vi "Test Sequence.vi"(0 "FeedBack Channel":string[](array[string])=["fgdgfvcbc", "vnfhgjkn", "21354682"], 1 "Test Name":string, 2 "Steps":T1(array[cluster])) -> (6 "Emergency":bool, 7 "Out":i32, 8 "Condition":bool)   [LabVIEW 2015]
uses:
  <vilib>/Utility/error.llb/whitespace.ctl
  Galobal variable_TI.vi
  Project Setup/Globle Variable/GR_Servo.vi
  <vilib>/Instr/_visa.llb/VISA Configure Serial Port (Instr).vi
panel:
  out "error out 2":errorcluster
  in  "value":bool
  out "read buffer":string
  out "error out":errorcluster
  out "Wait/Poll (ms)":u32
  out "Channels (Out)":i32[](array[numeric])
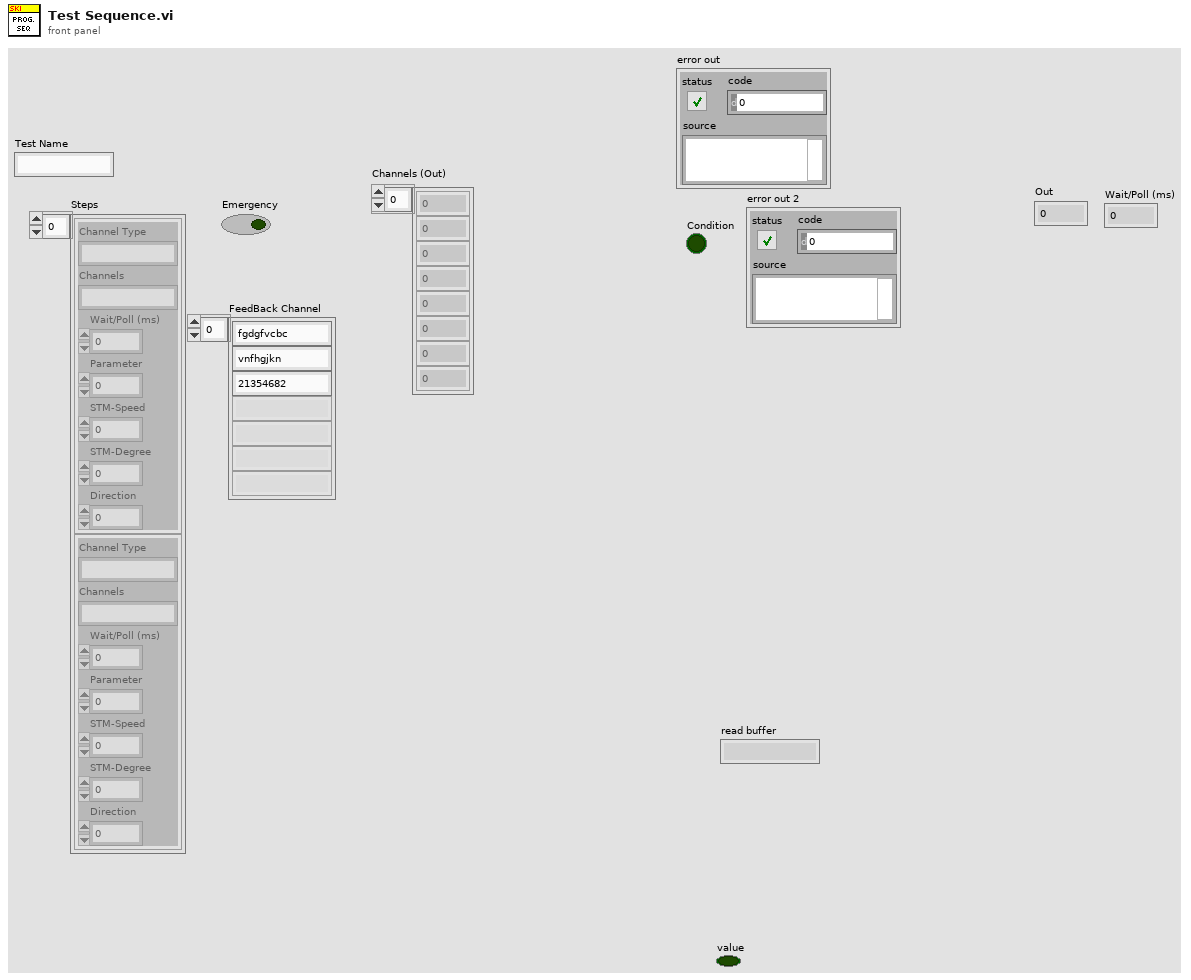
[diagram p1: front panel]
types:
  T1 = cluster{"Channel Type":string, "Channels":string, "Wait/Poll (ms)":u32, "Parameter":u8, "STM-Speed":i32, "STM-Degree":u32, "Direction":u8}[]
  T2 = cluster{"Emergency_1":bool, "Reset_2":bool, "Air Pressure_4":bool, "Safety Sensor_5":bool, "Safety Sensor_6":bool, "Barcode Rev rs_24":bool, "Clamp fwd rs_21":bool, "Servo Fault":bool, "Home _3":bool}
  T3 = cluster{"MIC ":refnum<visa-resource-name>, "baud rate MIC ":u32, "LCD ":refnum<visa-resource-name>, "baud rate_LCD":u32}
  T4 = cluster{"LVDT1Max(mm) AI0":dbl, "LVDT1Min (mm)AI0":dbl, "LVDT2Max(mm) AI1":dbl, "LVDT2Min(mm) AI1":dbl, "LVDT3Max(mm) AI2":dbl, "LVDT3Min(mm) AI2":dbl, "LVDT4Max(mm) AI3":dbl, "LVDT4Min(mm) AI3":dbl, "Model":string, "MIC Code":string}
  T5 = typedef "whitespace.ctl" = u16
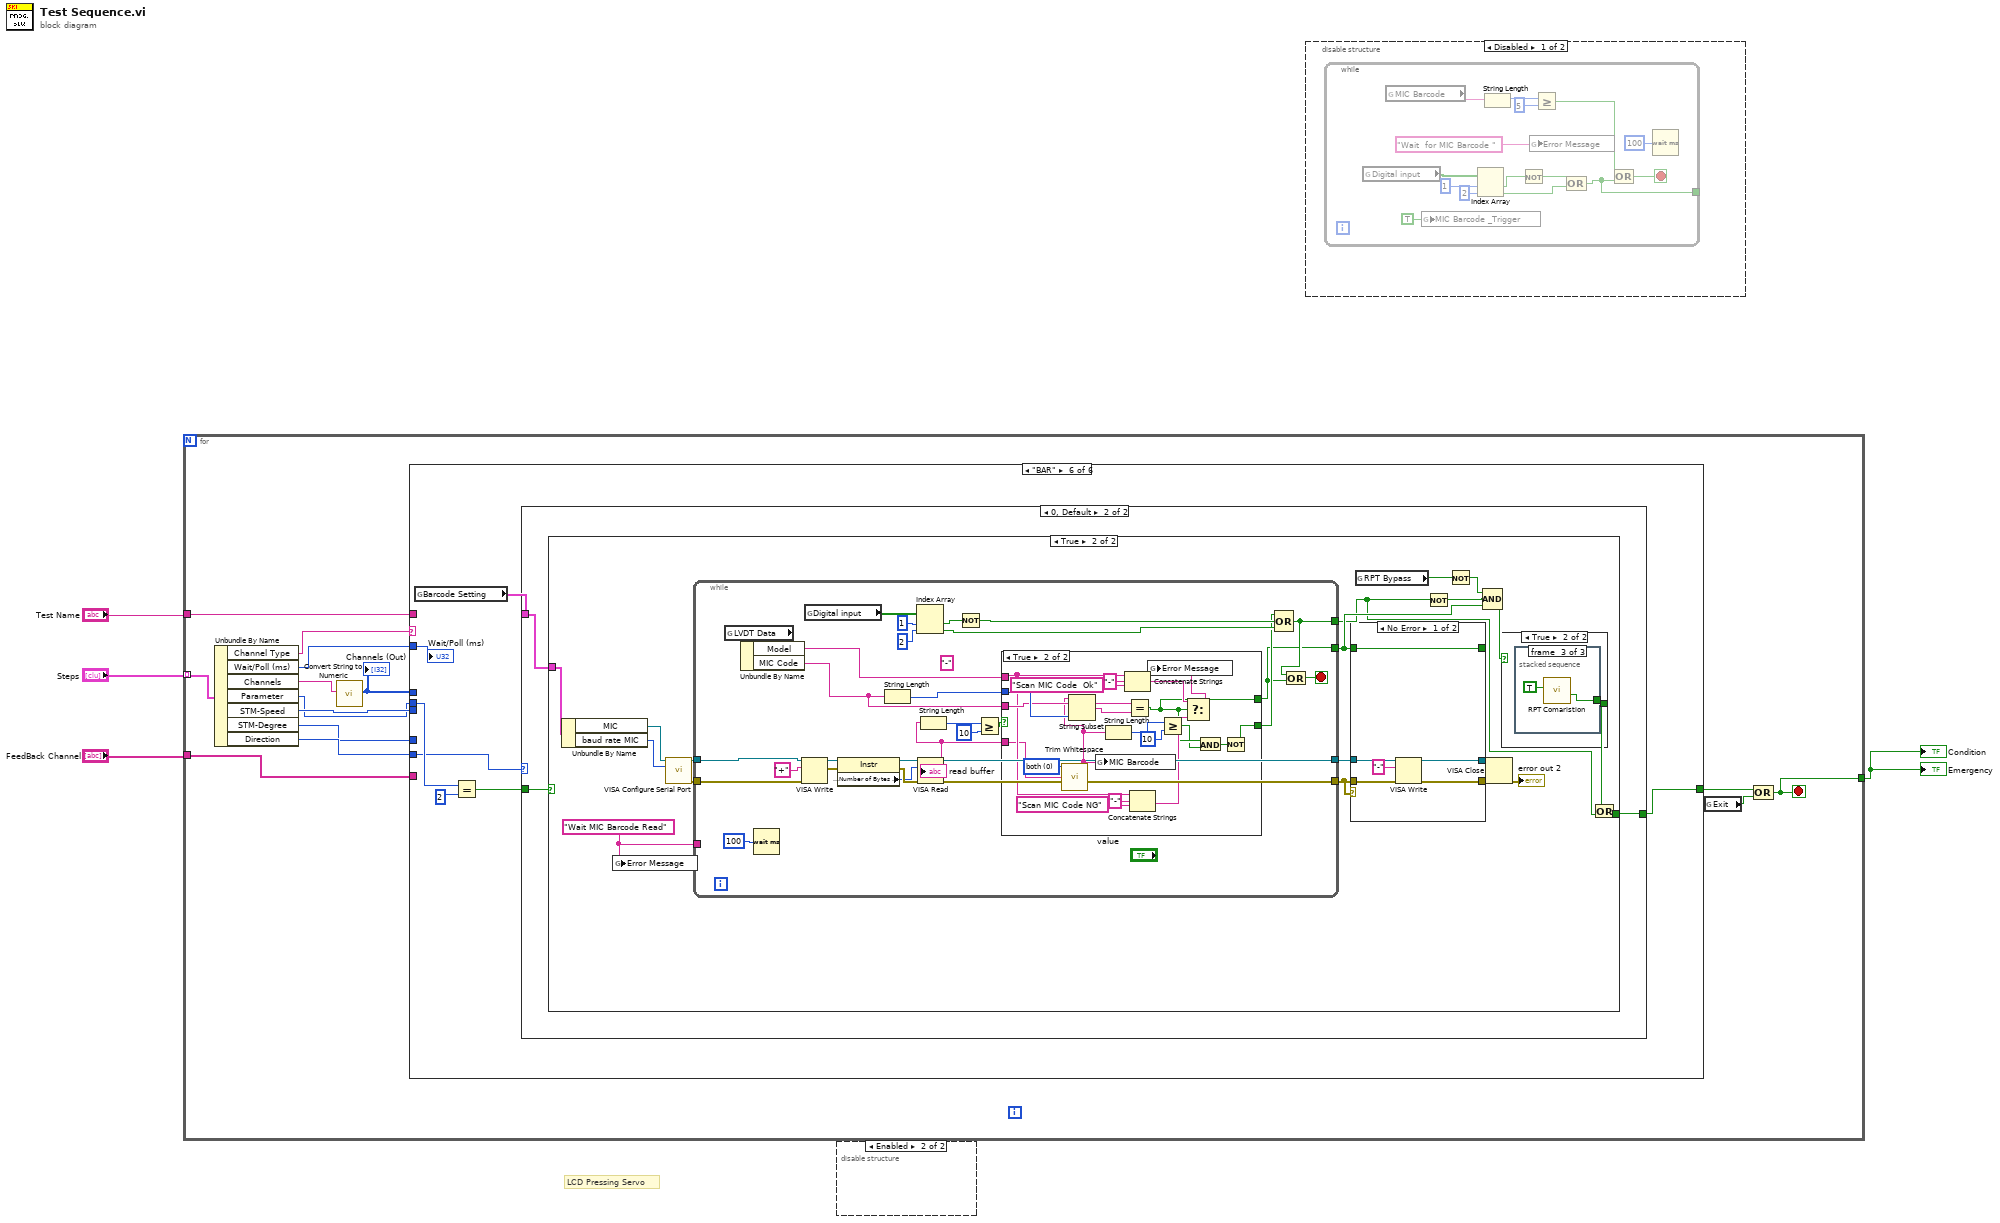
[diagram p0: block diagram]
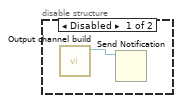
[diagram p3: hidden frame]
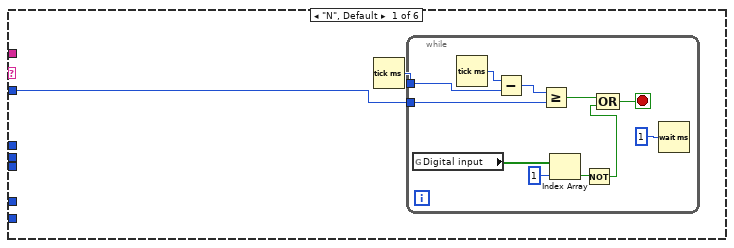
[diagram p4: hidden frame]
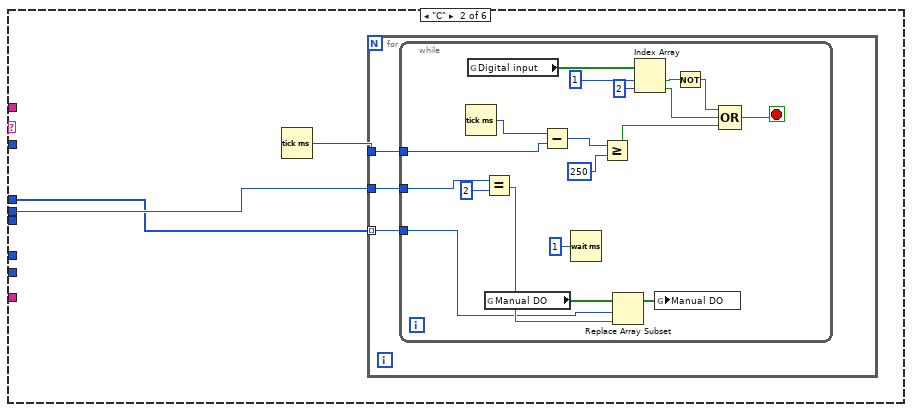
[diagram p5: hidden frame]
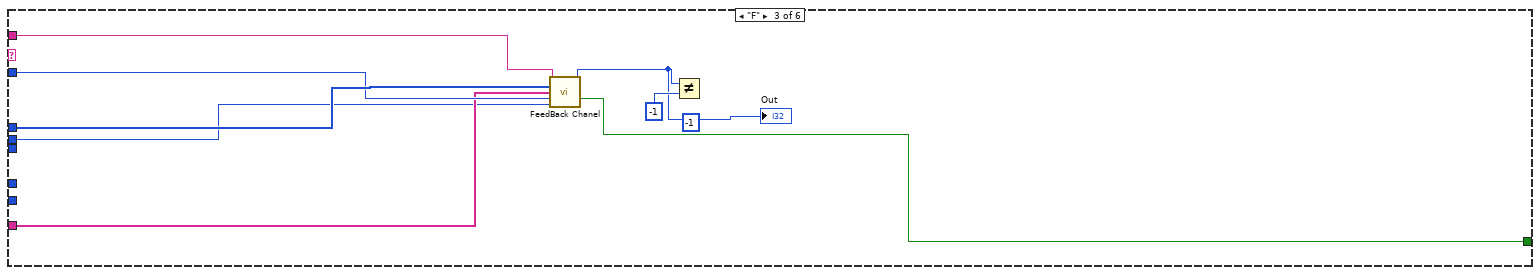
[diagram p6: hidden frame]
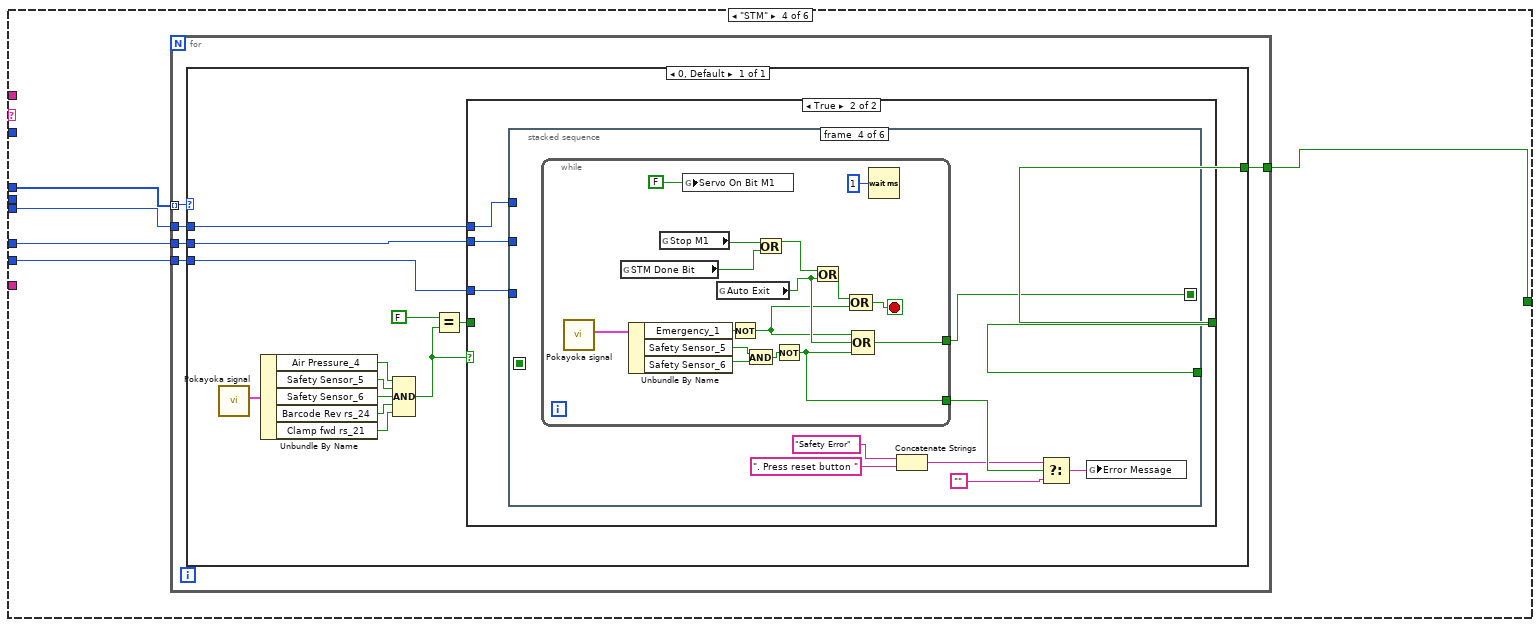
[diagram p7: hidden frame]
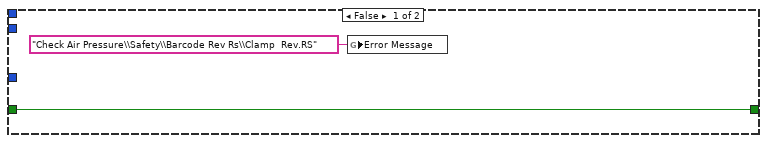
[diagram p8: hidden frame]
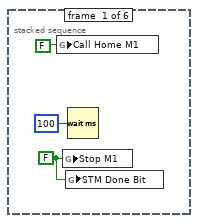
[diagram p9: hidden frame]
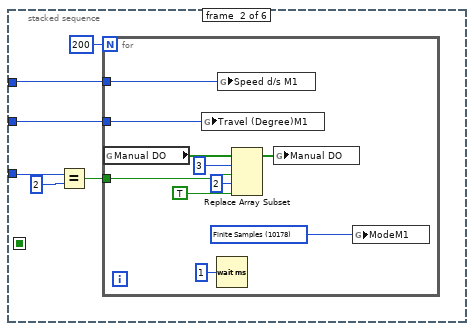
[diagram p10: hidden frame]
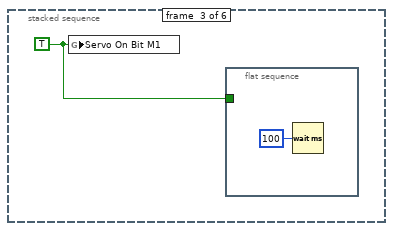
[diagram p11: hidden frame]
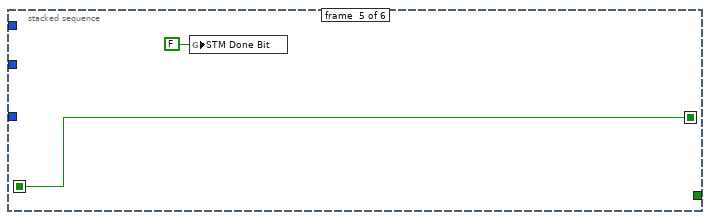
[diagram p12: hidden frame]
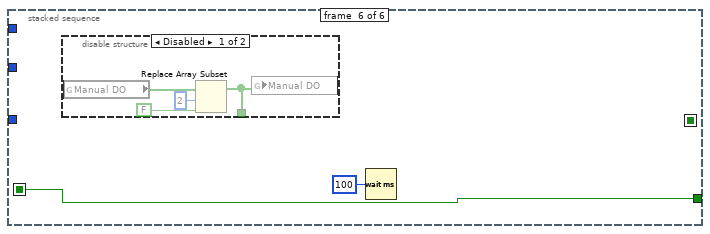
[diagram p13: hidden frame]
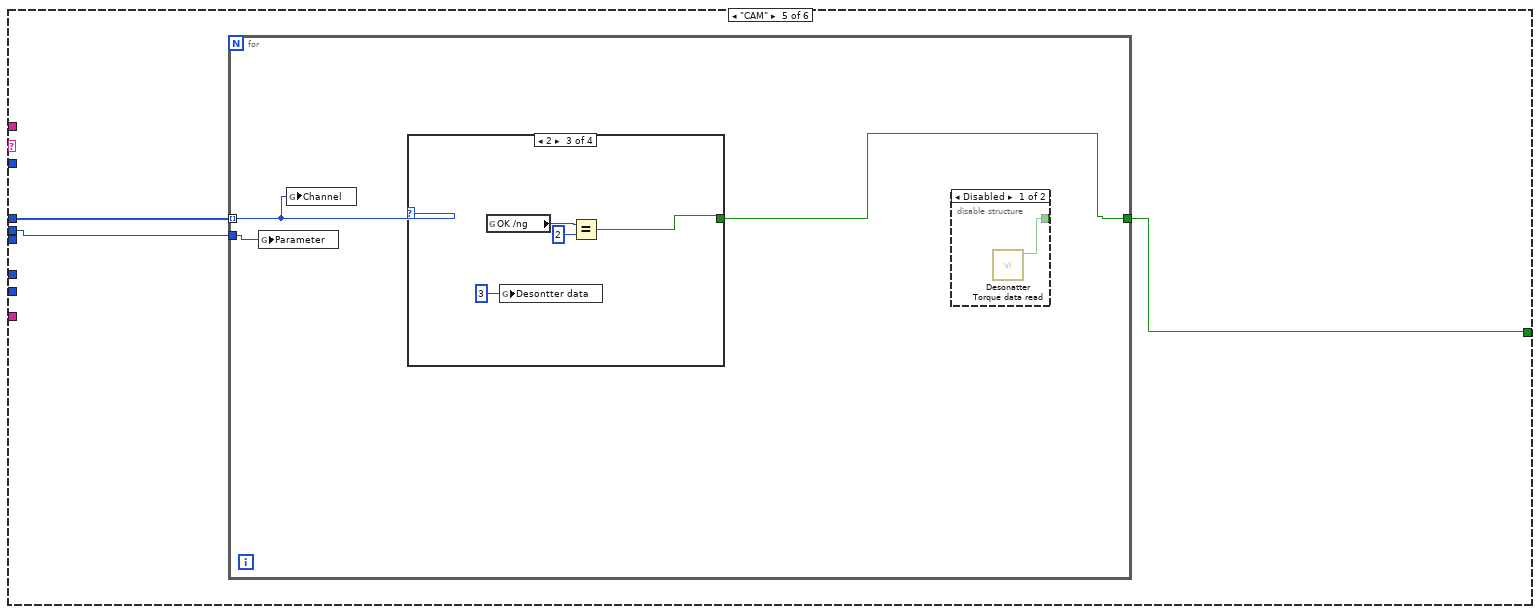
[diagram p15: hidden frame]
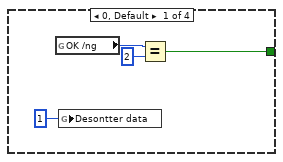
[diagram p17: hidden frame]
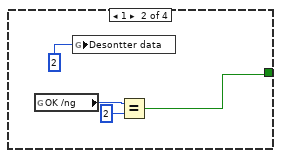
[diagram p18: hidden frame]
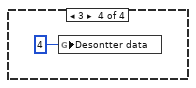
[diagram p19: hidden frame]
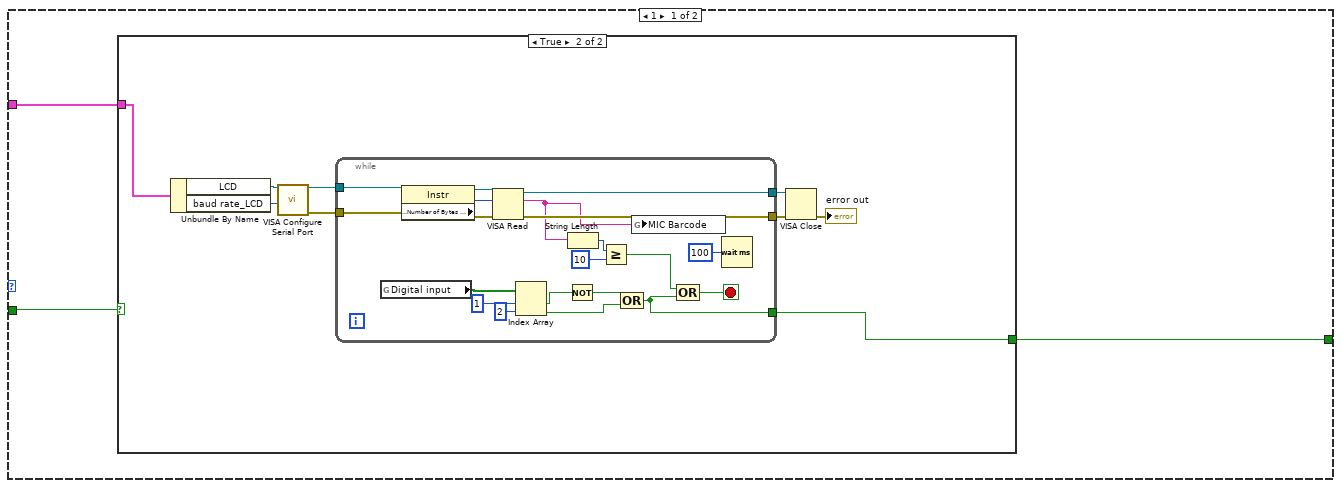
[diagram p20: hidden frame]
diagram:
  # "LCD Pressing Servo"
  n1 = for {
    tunnel: "Steps" -> [w18] mode=indexing
    tunnel: [w5] -> w1
    tunnel: "Test Name" -> [w13]
    tunnel: "FeedBack Channel" -> [w12]
    stop <- w5 stop-if-true
    n2 = Unbundle By Name(w18) -> ("Channel Type"=w17:string, "Wait/Poll (ms)"=w16:u32, "Channels"=w15:string, "Parameter"=w6:u8, "STM-Speed"=w8:i32, "STM-Degree"=w7:u32, "Direction"=w9:u8)
    n3 = call "Convert String to Numeric.vi"("Channels (A:B:C:D...) (In)"=w15) -> ("Channels (Out)"=w14:i32[])  [unwired: 9 in, 1 out]
    "Channels (Out)" <- w14
    n4 = case shown="\"BAR\"" w17 {
      tunnel: w16 -> [w19 _ w63 _ _ w172]
      tunnel: w14 -> [_ w32 w64 w69 w148 _]
      tunnel: w9 -> [_ _ _ w68 _ w167]
      tunnel: w13 -> [_ _ w62 _ _ _]
      tunnel: w12 -> [_ _ w61 _ _ _]
      tunnel: [_ _ w59 w65 w146 w168] -> w10
      tunnel: w8 -> [_ _ _ w67 _ _]
      tunnel: w7 -> [_ _ _ w66 _ _]
      tunnel: w6 -> [_ w34 w60 _ w147 w171]
      frame "N", Default {
        n5 = Tick Count (ms)() -> (millisecond timer value=w20:u32)
        n6 = while {
          tunnel: w20 -> [w30]
          tunnel: w19 -> [w25]
          stop <- w26 stop-if-true
          n7 = global read "Galobal variable_TI.vi" "Digital input"() -> (w24:bool[])
          n8 = Tick Count (ms)() -> (millisecond timer value=w31:u32)
          n9 = Subtract(x=w31, y=w30) -> (x-y=w29:u32)
          n10 = Greater Or Equal?(x=w29, y=w25) -> (x >= y?=w27:bool)
          n11 = Index Array(array=w24, index=1) -> (element=w22:bool)
          n12 = Not(x=w22) -> (.not. x?=w21:bool)
          n13 = Compound Arithmetic op=OR(w27, w21) -> (w26:bool)
          n14 = Wait (ms)(milliseconds to wait=u32 1) -> ()  [unwired: 1 out]
        }
      }
      frame "C" {
        n15 = Tick Count (ms)() -> (millisecond timer value=w33:u32)
        n16 = for {
          tunnel: w32 -> [w36] mode=indexing
          tunnel: w34 -> [w37]
          tunnel: w33 -> [w35]
          n17 = while {
            tunnel: w37 -> [w56]
            tunnel: w36 -> [w50]
            tunnel: w35 -> [w48]
            stop <- w45 stop-if-true
            n18 = Tick Count (ms)() -> (millisecond timer value=w49:u32)
            n19 = global read "Galobal variable_TI.vi" "Digital input"() -> (w44:bool[])
            n20 = Equal?(x=w56, y=u8 2) -> (x = y?=w51:bool)
            n21 = global read "Galobal variable_TI.vi" "Manual DO"() -> (w52:bool[])
            n22 = Subtract(x=w49, y=w48) -> (x-y=w47:u32)
            n23 = Wait (ms)(milliseconds to wait=u32 1) -> ()  [unwired: 1 out]
            n24 = Greater Or Equal?(x=w47, y=u32 250) -> (x >= y?=w38:bool)
            n25 = Replace Array Subset(array=w52, new element=w51, index=w50) -> (w53:bool[])
            n26 = Index Array(array=w44, index #1=1 ("index"), index #2=2 ("index")) -> (element #1=w42:bool, element #2=w39:bool)
            n27 = global write "Galobal variable_TI.vi" "Manual DO"(w53) -> ()
            n28 = Not(x=w42) -> (.not. x?=w40:bool)
            n29 = Compound Arithmetic op=OR(w40, w39, w38) -> (w45:bool)
          }
        }
      }
      frame "F" {
        (unwired) -1 ("Out")
        n30 = call "FeedBack Chanel.vi"("Test Name"=w62, "Channels (Int)"=w64, "FeedBack Channel"=w61, "Wait/Poll (ms)"=w63, "Parameter"=w60) -> ("Out"=w57:i32, "Exit"=w59:bool)  [unwired: 6 in, 3 out]
        "Out" <- w57
        n31 = Not Equal?(x=w57, y=-1) -> ()  [unwired: 1 out]
      }
      frame "STM" {
        n32 = for {
          tunnel: w69 -> [w74] mode=indexing
          tunnel: w68 -> [w73]
          tunnel: w67 -> [w72]
          tunnel: w66 -> [w71]
          tunnel: [w70] -> w65
          n33 = case shown="0, Default" w74 {
            tunnel: w73 -> [w85]
            tunnel: w72 -> [w87]
            tunnel: w71 -> [w86]
            tunnel: [w82] -> w70
            frame 0, Default {
              n34 = call "Pokayoka signal.vi"() -> ("output cluster"=w81:T2)  [unwired: 10 in, 1 out]
              n35 = Unbundle By Name(w81) -> ("Air Pressure_4"=w80:bool, "Safety Sensor_5"=w79:bool, "Safety Sensor_6"=w78:bool, "Barcode Rev rs_24"=w77:bool, "Clamp fwd rs_21"=w76:bool)
              n36 = Compound Arithmetic op=AND(w80, w79, w78, w77, w76) -> (w75:bool)
              n37 = Equal?(x=FALSE ("y"), y=w75) -> (x = y?=w83:bool)
              n38 = case shown="True" w75 {
                tunnel: w87 -> [_ w93]
                tunnel: w86 -> [_ w92]
                tunnel: w85 -> [_ w91]
                tunnel: [w89 w90] -> w82
                tunnel: w83 -> [w89 _]
                frame False {
                  n39 = global write "GR_Servo.vi" "Error Message"("Check Air Pressure\\Safety\\Barcode Rev Rs\\Clamp  Rev.RS" ("Error Message")) -> ()
                }
                frame True {
                  n40 = stacked-sequence {
                    seq-local: [_ _ _ w121 _ _] -> [_ _ _ _ w138 _]
                    seq-local: [_ _ _ _ w138 _] -> [_ _ _ _ _ w140]
                    tunnel: w92 -> [_ w102 _ _ _ _]
                    tunnel: w91 -> [_ w100 _ _ _ _]
                    tunnel: w93 -> [_ w98 _ _ _ _]
                    tunnel: [_ _ _ _ _ w140] -> w90
                    frame #0 {
                      w94 = FALSE ("Stop M1")
                      n41 = global write "Galobal variable_TI.vi" "Call Home M1"(FALSE ("Call Home M2")) -> ()
                      n42 = global write "Galobal variable_TI.vi" "Stop M1"(w94) -> ()
                      n43 = global write "Galobal variable_TI.vi" "STM Done Bit"(w94) -> ()
                      n44 = Wait (ms)(milliseconds to wait=u32 100) -> ()  [unwired: 1 out]
                    }
                    frame #1 {
                      n45 = Equal?(x=w100, y=u8 2) -> (x = y?=w99:bool)
                      n46 = for {
                        N: 200 -> [_]
                        tunnel: w102 -> [w112]
                        tunnel: w99 -> [w110]
                        tunnel: w98 -> [w108]
                        w111 = 10178 items=["Finite Samples"=10178, "Continuous Samples"=10123, "Hardware Timed Single Point"=12522] ("ModeM1")
                        n47 = global read "Galobal variable_TI.vi" "Manual DO"() -> (w106:bool[])
                        n48 = global write "GR_Servo.vi" "Travel (Degree)M1"(w112) -> ()
                        n49 = Wait (ms)(milliseconds to wait=u32 1) -> ()  [unwired: 1 out]
                        n50 = global write "GR_Servo.vi" "Speed d/s M1"(w108) -> ()
                        n51 = Replace Array Subset(array=w106, new element #1=w110, index #1=3 ("index"), new element #2=TRUE ("new element/subarray"), index #2=2 ("index")) -> (w109:bool[])
                        n52 = global write "Galobal variable_TI.vi" "Manual DO"(w109) -> ()
                        n53 = global write "GR_Servo.vi" "ModeM1"(w111) -> ()
                      }
                    }
                    frame #2 {
                      w113 = TRUE ("Servo On Bit")
                      n54 = global write "GR_Servo.vi" "Servo On Bit M1"(w113) -> ()
                      n55 = flat-sequence {
                        tunnel: w113 -> [_]
                        frame #0 {
                          n56 = Wait (ms)(milliseconds to wait=u32 100) -> ()  [unwired: 1 out]
                        }
                      }
                    }
                    frame #3 {
                      n57 = while {
                        tunnel: [w127] -> w121
                        tunnel: [w122] -> w119
                        stop <- w130 stop-if-true
                        n58 = call "Pokayoka signal.vi"() -> ("output cluster"=w132:T2)  [unwired: 10 in, 1 out]
                        n59 = global read "Galobal variable_TI.vi" "STM Done Bit"() -> (w135:bool)
                        n60 = Unbundle By Name(w132) -> ("Emergency_1"=w129:bool, "Safety Sensor_5"=w125:bool, "Safety Sensor_6"=w124:bool)
                        n61 = global read "Galobal variable_TI.vi" "Stop M1"() -> (w136:bool)
                        n62 = global write "GR_Servo.vi" "Servo On Bit M1"(FALSE ("Servo On Bit")) -> ()
                        n63 = global read "Galobal variable_TI.vi" "Auto Exit"() -> (w128:bool)
                        n64 = Not(x=w129) -> (.not. x?=w126:bool)
                        n65 = And(x=w125, y=w124) -> (x .and. y?=w123:bool)
                        n66 = Or(x=w136, y=w135) -> (x .or. y?=w133:bool)
                        n67 = Not(x=w123) -> (.not. x?=w122:bool)
                        n68 = Or(x=w133, y=w128) -> (x .or. y?=w131:bool)
                        n69 = Compound Arithmetic op=OR(w131, w126) -> (w130:bool)
                        n70 = Compound Arithmetic op=OR(w126, w128, w122) -> (w127:bool)
                        n71 = Wait (ms)(milliseconds to wait=u32 1) -> ()  [unwired: 1 out]
                      }
                      n72 = Concatenate Strings("Safety Error" ("string"), ". Press reset button ") -> (w117:string)
                      n73 = Select(t=w117, s=w119, f="") -> (s? t:f=w120:string)
                      n74 = global write "GR_Servo.vi" "Error Message"(w120) -> ()
                    }
                    frame #4 {
                      n75 = global write "Galobal variable_TI.vi" "STM Done Bit"(FALSE ("STM Done Bit LCD Pressing")) -> ()
                    }
                    frame #5 {
                      n76 = disable-structure shown="Disabled" {
                        disable-tunnel: [w142 _] -> _
                        frame Disabled {
                          n77 = global read "Galobal variable_TI.vi" "Manual DO"() -> (w145:bool[])
                          n78 = Replace Array Subset(array=w145, new element=FALSE ("new element/subarray"), index=2) -> (w142:bool[])
                          n79 = global write "Galobal variable_TI.vi" "Manual DO"(w142) -> ()
                        }
                        frame Enabled {
                        }
                      }
                      n80 = Wait (ms)(milliseconds to wait=u32 100) -> ()  [unwired: 1 out]
                    }
                  }
                }
              }
            }
          }
        }
      }
      frame "CAM" {
        n81 = for {
          tunnel: w148 -> [w151] mode=indexing
          tunnel: w147 -> [w150]
          tunnel: [w149] -> w146
          n82 = global write "Galobal variable_TI.vi" "Parameter"(w150) -> ()
          n83 = global write "Galobal variable_TI.vi" "Channel"(w151) -> ()
          n84 = case shown="2" w151 {
            tunnel: [w153 w157 w161 _] -> w149
            frame 0, Default {
              n85 = global read "Galobal variable_TI.vi" "OK /ng"() -> (w155:i32)
              n86 = global write "Galobal variable_TI.vi" "Desontter data"(1 ("Desontter data")) -> ()
              n87 = Equal?(x=w155, y=2) -> (x = y?=w153:bool)
            }
            frame 1 {
              n88 = global read "Galobal variable_TI.vi" "OK /ng"() -> (w159:i32)
              n89 = global write "Galobal variable_TI.vi" "Desontter data"(2 ("Desontter data")) -> ()
              n90 = Equal?(x=w159, y=2) -> (x = y?=w157:bool)
            }
            frame 2 {
              n91 = global read "Galobal variable_TI.vi" "OK /ng"() -> (w163:i32)
              n92 = global write "Galobal variable_TI.vi" "Desontter data"(3 ("Desontter data")) -> ()
              n93 = Equal?(x=w163, y=2) -> (x = y?=w161:bool)
            }
            frame 3 {
              n94 = global write "Galobal variable_TI.vi" "Desontter data"(4 ("Desontter data")) -> ()
            }
          }
          n95 = disable-structure shown="Disabled" {
            disable-tunnel: [w152 _] -> _
            frame Disabled {
              n96 = call "Desonatter Torque data read.vi"() -> ("Result"=w152:bool)  [unwired: 9 in, 2 out]
            }
            frame Enabled {
            }
          }
        }
      }
      frame "BAR" {
        n97 = global read "Galobal variable_TI.vi" "Barcode Setting"() -> (w166:T3)
        n98 = Equal?(x=w171, y=u8 2) -> (x = y?=w169:bool)
        n99 = case shown="0, Default" w167 {
          tunnel: w169 -> [w175 w208]
          tunnel: w166 -> [w174 w207]
          tunnel: [w173 w206] -> w168
          frame 1 {
            n100 = case shown="True" w175 {
              tunnel: w174 -> [_ w185]
              tunnel: [FALSE w177] -> w173
              frame False {
              }
              frame True {
                n101 = Unbundle By Name(w185) -> ("LCD"=w184:refnum<visa-resource-name>, "baud rate_LCD"=w183:u32)
                n102 = call-poly "VISA Configure Serial Port"("VISA resource name"=w184, "baud rate (9600)"=w183) -> ("VISA resource name out"=w182:refnum<visa-resource-name>, "error out"=w181:errorcluster)  [unwired: 12 in]
                n103 = while {
                  tunnel: w182 -> [w204]
                  tunnel: w181 -> [w205]
                  tunnel: [w198] -> w180
                  tunnel: [w197] -> w179
                  tunnel: [w187] -> w177
                  stop <- w189 stop-if-true
                  n104 = global read "Galobal variable_TI.vi" "Digital input"() -> (w196:bool[])
                  n105 = property class="Instr"(reference=w204, error in=w205) -> (reference out=w203:refnum<visa-resource-name>, error out=w202:errorcluster, "Serial Settings:Number of Bytes at Serial Port"=w201:u32)
                  n106 = VISA Read(VISA resource name=w203, byte count=w201, error in (no error)=w202) -> (VISA resource name out=w198:refnum<visa-resource-name>, read buffer=w186:string, error out=w197:errorcluster)  [unwired: 1 out]
                  n107 = Index Array(array=w196, index #1=1 ("index"), index #2=2 ("index")) -> (element #1=w193:bool, element #2=w191:bool)
                  n108 = Not(x=w193) -> (.not. x?=w192:bool)
                  n109 = String Length(string=w186) -> (length=w200:i32)
                  n110 = Greater Or Equal?(x=w200, y=10) -> (x >= y?=w190:bool)
                  n111 = Compound Arithmetic op=OR(w192, w191) -> (w187:bool)
                  n112 = global write "Galobal variable_TI.vi" "MIC Barcode"(w186) -> ()
                  n113 = Compound Arithmetic op=OR(w190, w187) -> (w189:bool)
                  n114 = Wait (ms)(milliseconds to wait=u32 100) -> ()  [unwired: 1 out]
                }
                n115 = VISA Close(VISA resource name=w180, error in (no error)=w179) -> (error out=→"error out":errorcluster)
              }
            }
          }
          frame 0, Default {
            n116 = case shown="True" w208 {
              tunnel: w207 -> [_ w222]
              tunnel: [FALSE w211] -> w206
              frame False {
                # "barcode bypass"
              }
              frame True {
                w218 = "Wait MIC Barcode Read"
                n117 = Unbundle By Name(w222) -> ("MIC"=w221:refnum<visa-resource-name>, "baud rate MIC"=w220:u32)
                n118 = global write "GR_Servo.vi" "Error Message"(w218) -> ()
                n119 = call-poly "VISA Configure Serial Port"("VISA resource name"=w221, "baud rate (9600)"=w220) -> ("VISA resource name out"=w228:refnum<visa-resource-name>, "error out"=w227:errorcluster)  [unwired: 12 in]
                n120 = while {
                  tunnel: w228 -> [w259]
                  tunnel: w227 -> [w258]
                  tunnel: [w268] -> w226
                  tunnel: [w267] -> w224
                  tunnel: w218 -> [_]
                  tunnel: [w245] -> w216
                  tunnel: [w246] -> w210
                  stop <- w252 stop-if-true
                  (unwired) "-" ("string")
                  n121 = global read "Galobal variable_TI.vi" "LVDT Data"() -> (w247:T4)
                  n122 = Unbundle By Name(w247) -> ("Model"=w251:string, "MIC Code"=w249:string)
                  n123 = Wait (ms)(milliseconds to wait=u32 100) -> ()  [unwired: 1 out]
                  n124 = VISA Write(VISA resource name=w259, write buffer="+", error in (no error)=w258) -> (VISA resource name out=w256:refnum<visa-resource-name>, error out=w257:errorcluster)  [unwired: 1 out]
                  n125 = global read "Galobal variable_TI.vi" "Digital input"() -> (w266:bool[])
                  n126 = property class="Instr"(reference=w256, error in=w257) -> (reference out=w273:refnum<visa-resource-name>, error out=w272:errorcluster, "Serial Settings:Number of Bytes at Serial Port"=w271:u32)
                  n127 = String Length(string=w249) -> (length=w250:i32)
                  n128 = Index Array(array=w266, index #1=1 ("index"), index #2=2 ("index")) -> (element #1=w263:bool, element #2=w261:bool)
                  n129 = VISA Read(VISA resource name=w273, byte count=w271, error in (no error)=w272) -> (VISA resource name out=w268:refnum<visa-resource-name>, read buffer=w254:string, error out=w267:errorcluster)  [unwired: 1 out]
                  "read buffer" <- w254
                  n130 = String Length(string=w254) -> (length=w270:i32)
                  n131 = Not(x=w263) -> (.not. x?=w262:bool)
                  n132 = Greater Or Equal?(x=w270, y=10) -> (x >= y?=w253:bool)
                  n133 = case shown="True" w253 {
                    tunnel: w254 -> [_ w278]
                    tunnel: w251 -> [_ w287]
                    tunnel: w250 -> [_ w294]
                    tunnel: w249 -> [_ w293]
                    tunnel: [FALSE w282] -> w245
                    tunnel: [FALSE w279] -> w248
                    frame False {
                    }
                    frame True {
                      w277 = T5 0 items=["both", "start of string", "end of string"] ("location (both)")
                      n134 = call <vilib>:"Trim Whitespace.vi"("string"=w278, "location (both)"=w277) -> ("trimmed string"=w276:string)
                      n135 = String Subset(string=w276, length (rest)=w294) -> (substring=w292:string)  [unwired: 1 in]
                      n136 = global write "Galobal variable_TI.vi" "MIC Barcode"(w276) -> ()
                      n137 = String Length(string=w276) -> (length=w283:i32)
                      n138 = Concatenate Strings(w287, "-" ("string"), "Scan MIC Code  Ok" ("string")) -> (w290:string)
                      n139 = Equal?(x=w293, y=w292) -> (x = y?=w282:bool)
                      n140 = Concatenate Strings(w287, "-" ("string"), "Scan MIC Code NG" ("string")) -> (w286:string)
                      n141 = Greater Or Equal?(x=w283, y=10) -> (x >= y?=w281:bool)
                      n142 = Select(t=w290, s=w282, f=w286) -> (s? t:f=w285:string)
                      n143 = global write "GR_Servo.vi" "Error Message"(w285) -> ()
                      n144 = And(x=w282, y=w281) -> (x .and. y?=w280:bool)
                      n145 = Not(x=w280) -> (.not. x?=w279:bool)
                    }
                  }
                  n146 = Compound Arithmetic op=OR(w248, w262, w261) -> (w246:bool)
                  n147 = Compound Arithmetic op=OR(w246, w245) -> (w252:bool)
                }
                n148 = case shown="No Error" w224 {
                  tunnel: w226 -> [w240 w244]
                  tunnel: [w239 w244] -> w225
                  tunnel: [w237 errorcluster {"status"=FALSE, "code"=0, "source"=""} ("error out")] -> w223
                  tunnel: w224 -> [w238 _]
                  tunnel: [w236 w242] -> _
                  tunnel: w216 -> [w236 w242]
                  frame No Error {
                    n149 = VISA Write(VISA resource name=w240, write buffer="-", error in (no error)=w238) -> (VISA resource name out=w239:refnum<visa-resource-name>, error out=w237:errorcluster)  [unwired: 1 out]
                  }
                  frame Error {
                  }
                }
                n150 = global read "Galobal variable_TI.vi" "RPT Bypass"() -> (w215:bool)
                n151 = Not(x=w210) -> (.not. x?=w213:bool)
                n152 = Not(x=w215) -> (.not. x?=w212:bool)
                n153 = Compound Arithmetic op=AND(w212, w213, w216) -> (w214:bool)
                n154 = VISA Close(VISA resource name=w225, error in (no error)=w223) -> (error out=→"error out 2":errorcluster)
                n155 = case shown="True" w214 {
                  tunnel: [FALSE ("Fail") w231] -> w217
                  frame False {
                    n156 = global write "Galobal variable_TI.vi" "Rework Bit"(TRUE ("Rework Bit")) -> ()
                  }
                  frame True {
                    n157 = stacked-sequence {
                      tunnel: [_ _ w235] -> w231
                      frame #0 {
                        n158 = global write "Galobal variable_TI.vi" "Rpt Read"(TRUE ("Rpt Read")) -> ()
                      }
                      frame #1 {
                        n159 = Wait (ms)(milliseconds to wait=u32 200) -> ()  [unwired: 1 out]
                      }
                      frame #2 {
                        n160 = call "RPT Comaristion.vi"("True"=TRUE) -> ("Fail"=w235:bool)  [unwired: 10 in]
                      }
                    }
                  }
                }
                n161 = Or(x=w217, y=w210) -> (x .or. y?=w211:bool)
              }
            }
          }
        }
        "Wait/Poll (ms)" <- w172
      }
    }
    n162 = global read "Galobal variable_TI.vi" "Exit"() -> (w11:bool)
    n163 = Compound Arithmetic op=OR(w10, w11) -> (w5:bool)
  }
  "Emergency" <- w1
  "Condition" <- w1
  n164 = disable-structure shown="Enabled" {
    frame Disabled {
      n165 = call "Output channel build.vi"() -> ("Output channel"=w296:refnum<notifier>)  [unwired: 11 in]
      n166 = Send Notification(notifier=w296) -> ()  [unwired: 2 in, 2 out]
    }
    frame Enabled {
    }
  }
  n167 = disable-structure shown="Disabled" {
    frame Disabled {
      n168 = while {
        tunnel: [w303] -> _
        stop <- w305 stop-if-true
        n169 = global read "Galobal variable_TI.vi" "Digital input"() -> (w311:bool[])
        n170 = global read "Galobal variable_TI.vi" "MIC Barcode"() -> (w302:string)
        n171 = global write "Galobal variable_TI.vi" "MIC Barcode _Trigger"(TRUE ("MIC Barcode _Trigger")) -> ()
        n172 = Index Array(array=w311, index #1=1 ("index"), index #2=2 ("index")) -> (element #1=w308:bool, element #2=w306:bool)
        n173 = String Length(string=w302) -> (length=w301:i32)
        n174 = Not(x=w308) -> (.not. x?=w307:bool)
        n175 = global write "GR_Servo.vi" "Error Message"("Wait  for MIC Barcode ") -> ()
        n176 = Greater Or Equal?(x=w301, y=5) -> (x >= y?=w299:bool)
        n177 = Compound Arithmetic op=OR(w307, w306) -> (w303:bool)
        n178 = Compound Arithmetic op=OR(w299, w303) -> (w305:bool)
        n179 = Wait (ms)(milliseconds to wait=u32 100) -> ()  [unwired: 1 out]
      }
    }
    frame Enabled {
    }
  }
